vi "Add IntelliSense Control.vi"(0 "IntelliSenseStringControl":refnum<class "IntelliSenseStringControl.lvclass">) -> (1 "IntelliSenseStringControl":refnum<class "IntelliSenseStringControl.lvclass">, 3 "Added?":bool)   [LabVIEW 2016, in "StringIntelliSense.lvlib" / "IntelliSenseStringControl.lvclass"]
uses:
  IntelliSenseStringControl.lvclass
  StringMonitorUserData.vi
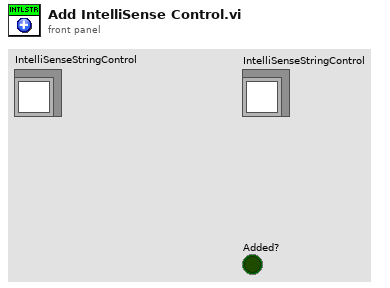
[diagram p1: front panel]
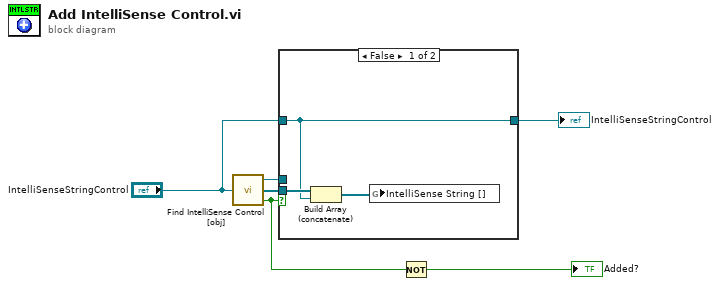
[diagram p0: block diagram]
diagram:
  n1 = call "Find IntelliSense Control [obj].vi"("IntelliSenseStringControl"="IntelliSenseStringControl") -> ("Found IntelliSenseStringControl"=w5:refnum<class "IntelliSenseStringControl.lvclass">, "Other IntelliSense String []"=w6:refnum<class "IntelliSenseStringControl.lvclass">[], "Found?"=w4:bool)
  n2 = case shown="False" w4 {
    tunnel: w6 -> [w9 _]
    tunnel: w5 -> [_ w10]
    tunnel: "IntelliSenseStringControl" -> [w7 _]
    tunnel: [w7 w10] -> w1
    frame False {
      n3 = Build Array (concatenate)(w9, w7) -> (w8:refnum<class "IntelliSenseStringControl.lvclass">[])
      n4 = global write "StringMonitorUserData.vi" "IntelliSense String []"(w8) -> ()
    }
    frame True {
    }
  }
  "IntelliSenseStringControl" <- w1
  n5 = Not(x=w4) -> (.not. x?=→"Added?":bool)
